vi "Within 10 Milliseconds.vi"(10 "milliseconds 2":u32 format="%.0x", 11 "milliseconds 1":u32 format="%.0x") -> (3 "within 10 ms":bool)   [LabVIEW 2013]
doc: "Compares two tick counts and reports whether they are within 10 ms of one another\n\n<b>DO NOT DISTRIBUTE THIS VI IN THE PRODUCT</b>\n\nAuthored by David Staab\nCopyright (c) 2015, Staab Engineering\nAll rights reserved.\n\nRedistribution and use in source and binary forms, with or without modification, are permitted provided that the following conditions are met:\n\n * Redistributions of source code must retain the above copyright notice, this list of conditions and the following disclaimer.\n * Redistributions in binary form must reproduce the above copyright notice, this list of conditions and the following disclaimer in the documentation and/or other materials provided with the distribution.\n * Neither the name of Staab Engineering nor the names of its contributors may be used to endorse or promote products derived from this software without specific prior written permission.\n\nTHIS SOFTWARE IS PROVIDED BY THE COPYRIGHT HOLDERS AND CONTRIBUTORS \"AS IS\" AND ANY EXPRESS OR IMPLIED WARRANTIES, INCLUDING, BUT NOT LIMITED TO, THE IMPLIED WARRANTIES OF MERCHANTABILITY AND FITNESS FOR A PARTICULAR PURPOSE ARE DISCLAIMED. IN NO EVENT SHALL THE COPYRIGHT OWNER OR CONTRIBUTORS BE LIABLE FOR ANY DIRECT, INDIRECT, INCIDENTAL, SPECIAL, EXEMPLARY, OR CONSEQUENTIAL DAMAGES (INCLUDING, BUT NOT LIMITED TO, PROCUREMENT OF SUBSTITUTE GOODS OR SERVICES; LOSS OF USE, DATA, OR PROFITS; OR BUSINESS INTERRUPTION) HOWEVER CAUSED AND ON ANY THEORY OF LIABILITY, WHETHER IN CONTRACT, STRICT LIABILITY, OR TORT (INCLUDING NEGLIGENCE OR OTHERWISE) ARISING IN ANY WAY OUT OF THE USE OF THIS SOFTWARE, EVEN IF ADVISED OF THE POSSIBILITY OF SUCH DAMAGE."
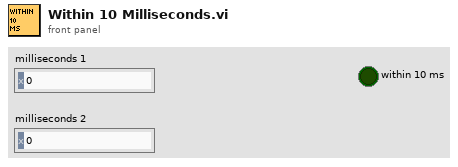
[diagram p1: front panel]
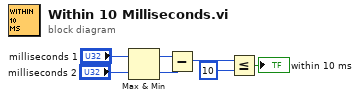
[diagram p0: block diagram]
diagram:
  n1 = Max & Min(x="milliseconds 1", y="milliseconds 2") -> (max(x,y)=w3:u32, min(x,y)=w1:u32)
  n2 = Subtract(x=w3, y=w1) -> (x-y=w7:u32)
  n3 = Less Or Equal?(x=w7, y=u32 10) -> (x <= y?=→"within 10 ms":bool)
